vi "Preflight Acquisition.vi"(4 "error in (no error)":errorcluster, 7 "pDataBuffer in":u16[](array[numeric])) -> (0 "error out":errorcluster, 2 "function return":i32, 3 "pDataBuffer out":u16[](array[numeric]))   [LabVIEW 2020, in "ThorConfocal.lvlib"]
doc: "long PreflightAcquisition(char * pDataBuffer);"
uses:
  ThorConfocal.lvlib
  C:/Program Files/Thorlabs/ThorImageLS 4.1/Modules_Native/ThorConfocal.dll
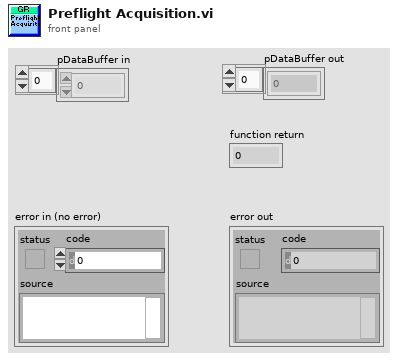
[diagram p1: front panel]
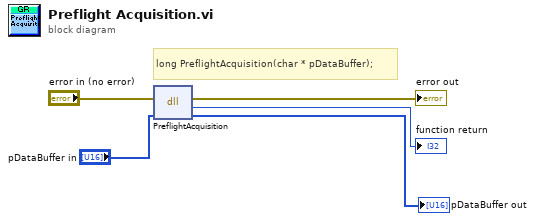
[diagram p0: block diagram]
diagram:
  # "long PreflightAcquisition(char * pDataBuffer);"
  n1 = dll-call lib="C:/Program Files/Thorlabs/ThorImageLS 4.1/Modules_Native/ThorConfocal.dll" fn="PreflightAcquisition"(error in="error in (no error)", "pDataBuffer"="pDataBuffer in") -> (error out=→"error out":errorcluster, "return type"=→"function return":i32, "pDataBuffer"=→"pDataBuffer out":u16[])  [unwired: 2 in, 1 out]
